vi "Calculate Mask Test Query.vi"(8 "error in":errorcluster, 10 "Calculation Channel":i32(ring) items=["Calc Channel 1", "Calc Channel 2", "Calc Channel 3", "Calc Channel 4"], 11 "Instrument Handle In":i32) -> (0 "error out":errorcluster, 1 "Lower Reference":i32, 2 "Source":i32, 3 "Instrument Handle Out":i32, 4 "Upper Reference":i32, 5 "Count":u32)   [LabVIEW 8.6, in "ZTScopeM.lvlib"]
doc: "Query the mask test settings of the selected calculation channel."
uses:
  ZTScopeM.lvlib
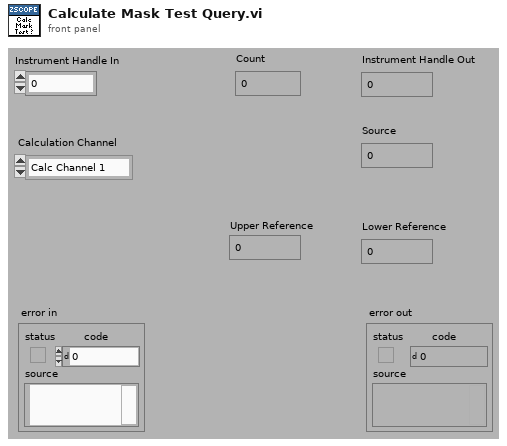
[diagram p1: front panel]
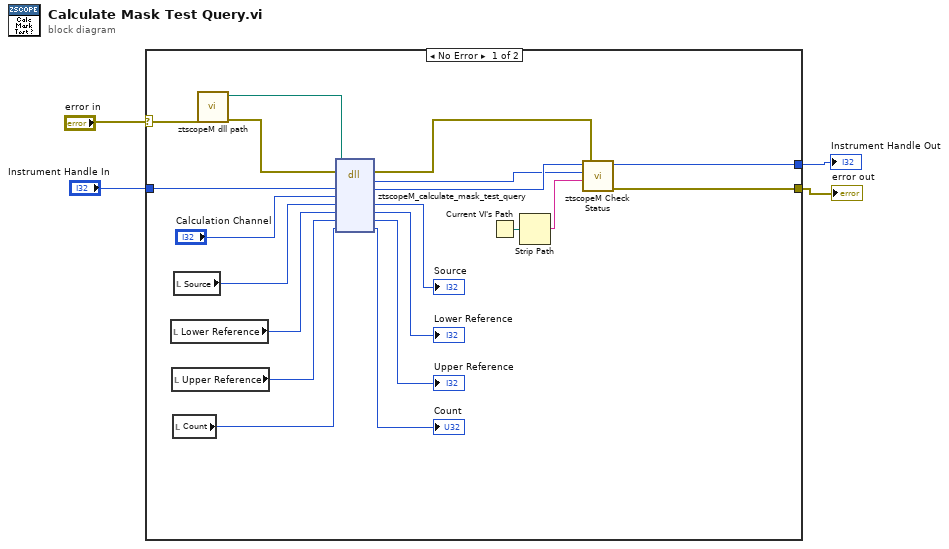
[diagram p0: block diagram]
diagram:
  n1 = case shown="No Error" "error in" {
    selector: "error in" -> [w8 w26]
    tunnel: [w12 w26] -> w1
    tunnel: "Instrument Handle In" -> [w24 w25]
    tunnel: [w11 w25] -> w2
    frame #0 {
      n2 = local read "Lower Reference"() -> (w20:i32)
      n3 = local read "Upper Reference"() -> (w18:i32)
      n4 = local read "Count"() -> (w9:u32)
      n5 = local read "Source"() -> (w22:i32)
      n6 = call "ztscopeM dll path.vi"("error in (no error)"=w8) -> ("error out"=w6:errorcluster, "<instrument>.dll path"=w7:path)  [unwired: 9 in]
      n7 = dll-call lib="C:/Program Files (x86)/National Instruments/LabVIEW 2013/instr.lib/ztscopem/ztscopeM.dll" fn="ztscopeM_calculate_mask_test_query"(path in=w7, error in=w6, "instrumentHandle"=w24, "calculationChannel"="Calculation Channel", "source"=w22, "lowerReference"=w20, "upperReference"=w18, "Count"=w9) -> (error out=w5:errorcluster, w13:i32, "instrumentHandle"=w14:i32, "source"=→"Source":i32, "lowerReference"=→"Lower Reference":i32, "upperReference"=→"Upper Reference":i32, "Count"=→"Count":u32)  [unwired: 2 in, 1 out]
      n8 = Current VI's Path() -> (path=w16:path)
      n9 = Strip Path(path=w16) -> (name=w15:string)  [unwired: 1 out]
      n10 = call "ztscopeM Check Status.vi"("error in"=w5, "name of VI"=w15, "status (return code)"=w13, "instrument handle in"=w14) -> ("error out"=w12:errorcluster, "instrument handle out"=w11:i32)  [unwired: 2 in]
    }
    frame #1 {
    }
  }
  "Instrument Handle Out" <- w2
  "error out" <- w1
